vi "Send Command Query (non-enum).vi"(8 "error in (no error)":errorcluster, 10 "Command":string, 11 "Gen 2 in":refnum<class "Gen 2.lvclass">) -> (0 "error out":errorcluster, 2 "Response":string, 3 "Gen 2 out":refnum<class "Gen 2.lvclass">)   [LabVIEW 2018, in "Gen 2.lvlib" / "Gen 2.lvclass"]
doc: "This Override is used to send a command to the targeted device and read the reponse\nNOTE: This Override was created to provide means to sends commands that are not part of the Command LIst.ctl whic was initially intended for Model H Laser (Kronos)"
uses:
  Gen 2.lvclass
  PPLs/Laser/Parent/Laser.lvlibp/Laser.lvclass
  C:/Projects/LabVIEW/PPLs/Laser/Parent/Laser.lvlibp/Laser.lvclass
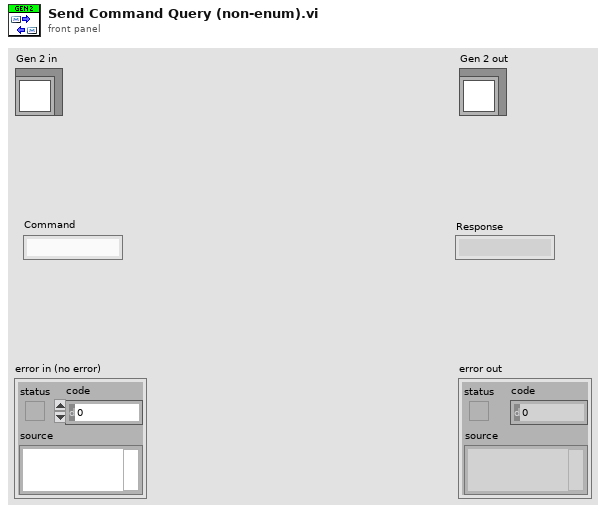
[diagram p1: front panel]
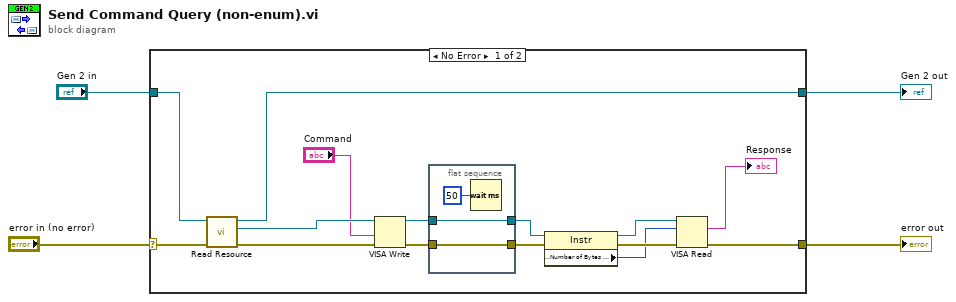
[diagram p0: block diagram]
diagram:
  n1 = case shown="No Error" "error in (no error)" {
    selector: "error in (no error)" -> [w18 w23]
    tunnel: "Gen 2 in" -> [w19 w24]
    tunnel: [w17 w24] -> w2
    tunnel: [w6 w23] -> w1
    frame No Error {
      n2 = call "Read Resource.vi"("error in (no error)"=w18, "Laser in"=w19) -> ("error out"=w16:errorcluster, "Resource"=w15:refnum<visa-resource-name>, "Laser out"=w17:refnum<class "Gen 2.lvclass">)  [unwired: 7 in]
      n3 = VISA Write(VISA resource name=w15, write buffer="Command", error in (no error)=w16) -> (VISA resource name out=w12:refnum<visa-resource-name>, error out=w13:errorcluster)  [unwired: 1 out]
      n4 = flat-sequence {
        tunnel: w13 -> [w20]
        tunnel: [w22] -> w11
        tunnel: w12 -> [w22]
        tunnel: [w20] -> w10
        frame #0 {
          n5 = Wait (ms)(milliseconds to wait=u32 50) -> ()  [unwired: 1 out]
        }
      }
      n6 = property class="Instr"(reference=w11, error in=w10) -> (reference out=w8:refnum<visa-resource-name>, error out=w9:errorcluster, "Serial Settings:Number of Bytes at Serial Port"=w7:u32)
      n7 = VISA Read(VISA resource name=w8, byte count=w7, error in (no error)=w9) -> (read buffer=→"Response":string, error out=w6:errorcluster)  [unwired: 2 out]
    }
    frame Error {
    }
  }
  "error out" <- w1
  "Gen 2 out" <- w2
